vi "waveform_moving_average.vi"(9 "window size":i32=5, 11 "waveform":waveform(dbl)) -> (3 "averaged waveform":waveform(dbl))   [LabVIEW 2017]
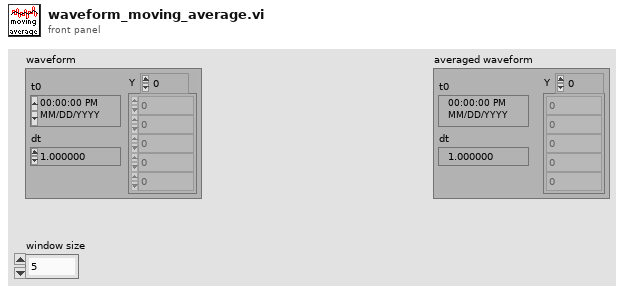
[diagram p1: front panel]
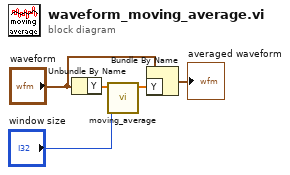
[diagram p0: block diagram]
diagram:
  n1 = Unbundle By Name("waveform") -> ("Y"=w5:dbl[])
  n2 = call "moving_average.vi"("window size"="window size", "X"=w5) -> ("averaged X"=w4:dbl[])  [unwired: 9 in]
  n3 = Bundle By Name(cluster="waveform", "Y"=w4) -> (→"averaged waveform":waveform(dbl))
